vi "Trimspace without return vs Trimspace with return.vi"() -> ()   [LabVIEW 2020]
panel:
  out "[\\t\\n\\r\\s]":string
  out "[\\t\\s]":string
  out "unit (ms) 2":dbl[](graph)
  out "inside 2":i32
  out "outside 2":i32
  out "inside":i32
  out "outside":i32
  out "unit (ms)":dbl[][](graph)
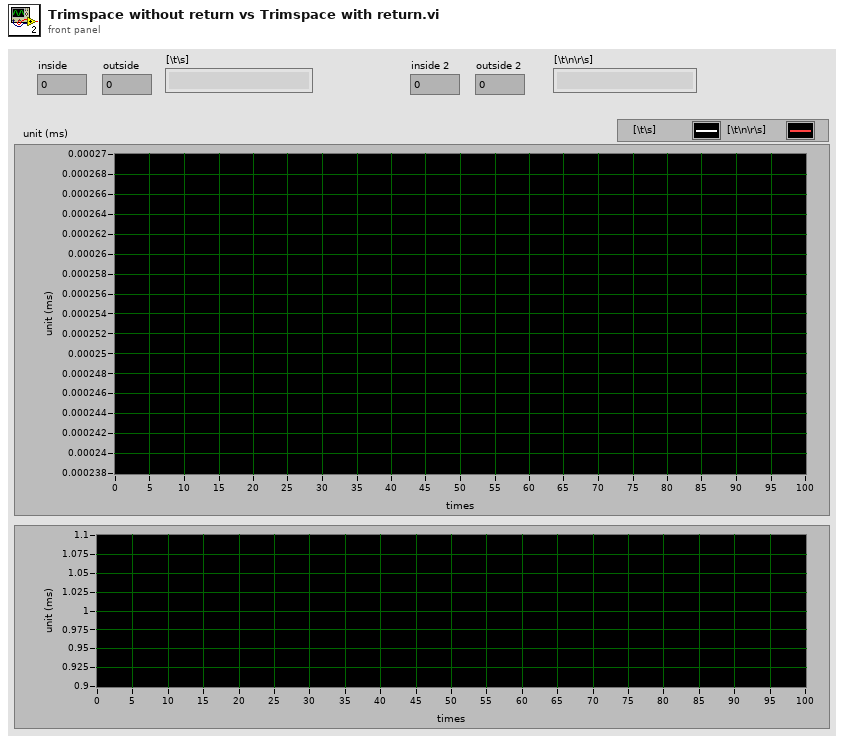
[diagram p1: front panel]
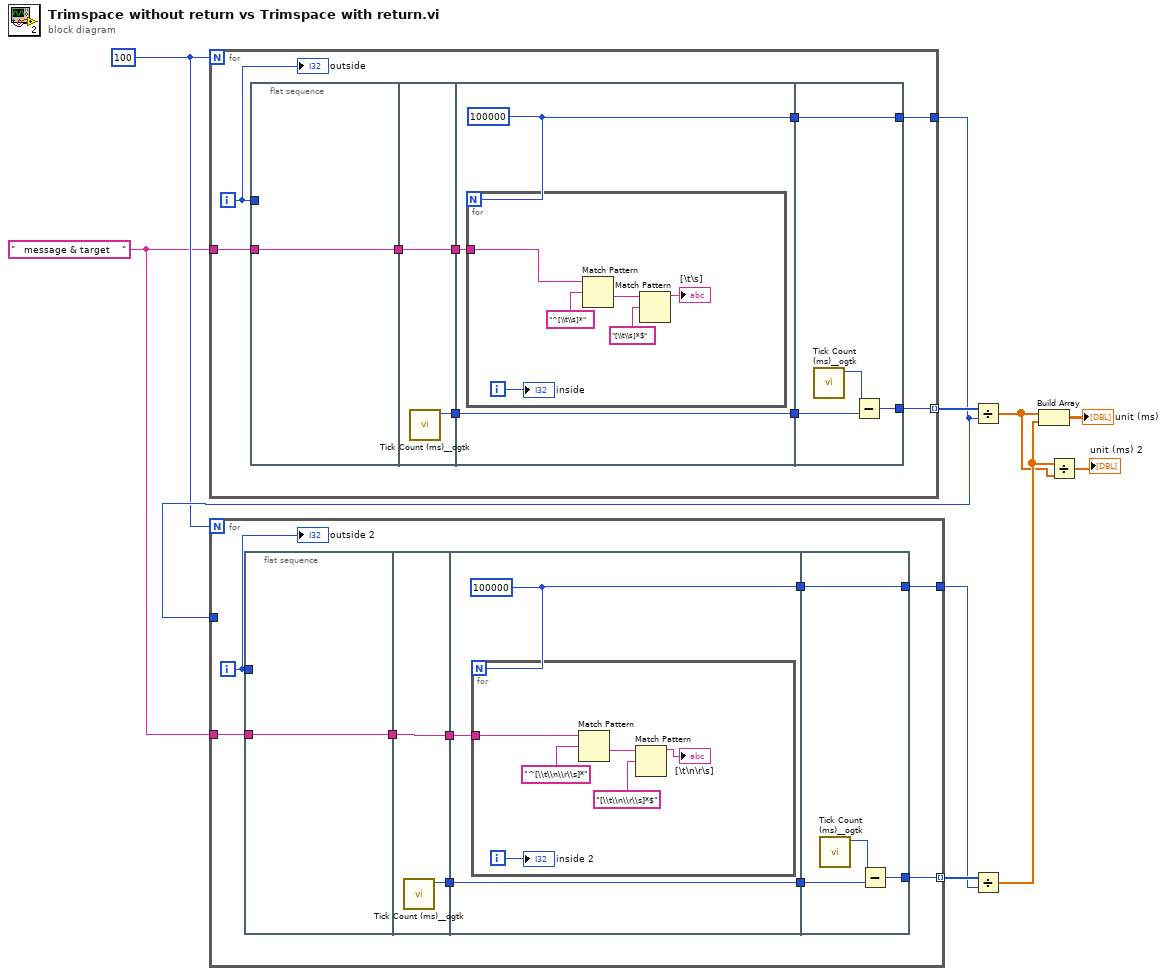
[diagram p0: block diagram]
diagram:
  w1 = "   message & target    " ("string")
  w5 = 100
  n1 = for {
    N: w5 -> [_]
    tunnel: [w17] -> w10 mode=indexing
    tunnel: [w16] -> w6
    tunnel: w1 -> [w11]
    i -> [w14]
    n2 = flat-sequence {
      tunnel: w14 -> [_]
      tunnel: [w20] -> w12
      tunnel: w11 -> [w20]
      tunnel: [w22] -> w19
      tunnel: [w21] -> w13
      tunnel: w12 -> [w21]
      tunnel: w19 -> [w25]
      tunnel: [w25] -> w18
      tunnel: [w24] -> w15
      tunnel: w13 -> [w23]
      tunnel: w18 -> [w34]
      tunnel: [w33] -> w17
      tunnel: [w32] -> w16
      tunnel: w15 -> [w32]
      frame #0 {
      }
      frame #1 {
        n3 = call <userlib>:"Tick Count (ms)__ogtk.vi"() -> ("millisecond timer value"=w22:u32)  [unwired: 10 in, 1 out]
      }
      frame #2 {
        w24 = 100000
        n4 = for {
          N: w24 -> [_]
          tunnel: w23 -> [w27]
          i -> [w31]
          n5 = Match Pattern(string=w27, regular expression="^[\\t\\s]*") -> (after substring=w28:string)  [unwired: 1 in, 3 out]
          n6 = Match Pattern(string=w28, regular expression="[\\t\\s]*$") -> (before substring=→"[\\t\\s]":string)  [unwired: 1 in, 3 out]
          "inside" <- w31
        }
      }
      frame #3 {
        n7 = call <userlib>:"Tick Count (ms)__ogtk.vi"() -> ("millisecond timer value"=w35:u32)  [unwired: 10 in, 1 out]
        n8 = Subtract(x=w35, y=w34) -> (x-y=w33:u32)
      }
    }
    "outside" <- w14
  }
  n9 = for {
    N: w5 -> [_]
    tunnel: [w42] -> w8 mode=indexing
    tunnel: [w41] -> w7
    tunnel: w6 -> [_]
    tunnel: w1 -> [w36]
    i -> [w39]
    n10 = flat-sequence {
      tunnel: w39 -> [_]
      tunnel: [w45] -> w37
      tunnel: w36 -> [w45]
      tunnel: [w47] -> w44
      tunnel: [w46] -> w38
      tunnel: w37 -> [w46]
      tunnel: w44 -> [w50]
      tunnel: [w50] -> w43
      tunnel: [w49] -> w40
      tunnel: w38 -> [w48]
      tunnel: w43 -> [w59]
      tunnel: [w58] -> w42
      tunnel: [w57] -> w41
      tunnel: w40 -> [w57]
      frame #0 {
      }
      frame #1 {
        n11 = call <userlib>:"Tick Count (ms)__ogtk.vi"() -> ("millisecond timer value"=w47:u32)  [unwired: 10 in, 1 out]
      }
      frame #2 {
        w49 = 100000
        n12 = for {
          N: w49 -> [_]
          tunnel: w48 -> [w51]
          i -> [w56]
          n13 = Match Pattern(string=w51, regular expression="^[\\t\\n\\r\\s]*") -> (after substring=w53:string)  [unwired: 1 in, 3 out]
          n14 = Match Pattern(string=w53, regular expression="[\\t\\n\\r\\s]*$") -> (before substring=→"[\\t\\n\\r\\s]":string)  [unwired: 1 in, 3 out]
          "inside 2" <- w56
        }
      }
      frame #3 {
        n15 = call <userlib>:"Tick Count (ms)__ogtk.vi"() -> ("millisecond timer value"=w60:u32)  [unwired: 10 in, 1 out]
        n16 = Subtract(x=w60, y=w59) -> (x-y=w58:u32)
      }
    }
    "outside 2" <- w39
  }
  n17 = Divide(x=w10, y=w6) -> (x/y=w3:dbl[])
  n18 = Divide(x=w8, y=w7) -> (x/y=w4:dbl[])
  n19 = Build Array(w3, w4) -> (→"unit (ms)":dbl[][])
  n20 = Divide(x=w4, y=w3) -> (x/y=→"unit (ms) 2":dbl[])
